vi "Copy VIP File sub.vi"(0 "CLI in":refnum<class "CLI.lvclass">, 5 "Array of created files":path[](array[path]), 11 "error in (no error)":errorcluster) -> (4 "CLI out":refnum<class "CLI.lvclass">, 15 "error out":errorcluster)   [LabVIEW 2023]
doc: "Copy VIP File sub.vi\n----------------------------------------------\nCopies the created *.vip file to the public user's documents folder\n\nInputs:\n---------------------\n- CLI in : LabVIEW Class Instance; \n- error in (no error) : Cluster; \n- Array of created files : 1DArrayOfPath; \n\nOutputs:\n---------------------\n- CLI out : LabVIEW Class Instance; \n- error out : Cluster; \n\n----------------------------------------------\n6/1/2021 nina\nZühlke Engineering AG\nCH-8952 Schlieren\nwww.zuehlke.com"
uses:
  <vilib>/Wiresmith Technology/G CLI/CLI Class/CLI.lvclass
panel:
  # "Connector Pane"
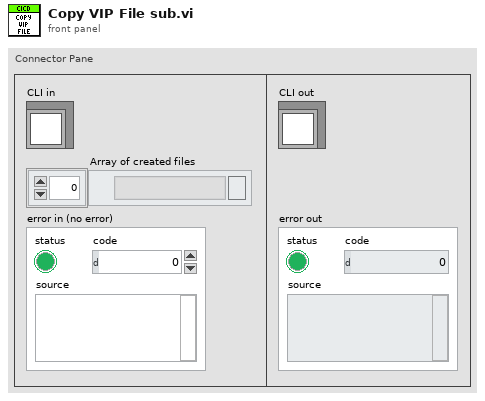
[diagram p1: front panel]
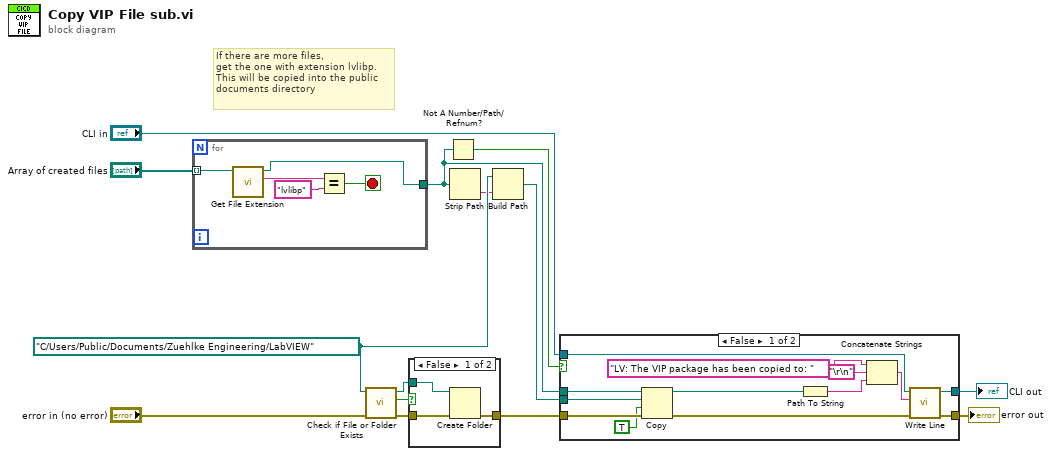
[diagram p0: block diagram]
diagram:
  w4 = path "C:/Users/Public/Documents/Zuehlke Engineering/LabVIEW" ("base path")
  # "If there are more files,\nget the one with extension lvlibp.\nThis will be copied into the public\ndocuments directory"
  n1 = for {
    tunnel: "Array of created files" -> [w19] mode=indexing
    tunnel: [w18] -> w12
    stop <- w15 stop-if-true
    n2 = call <vilib>:"Get File Extension.vi"("file"=w19) -> ("lowercase file extension"=w17:string, "dup file"=w18:path)  [unwired: 6 in, 3 out]
    n3 = Equal?(x=w17, y="lvlibp") -> (x = y?=w15:bool)
  }
  n4 = call <vilib>:"Check if File or Folder Exists.vi"("error in (no error)"="error in (no error)", "path"=w4) -> ("error out"=w6:errorcluster, "file or folder exists?"=w7:bool, "dup path"=w5:path)  [unwired: 7 in]
  n5 = case shown="False" w7 {
    tunnel: w5 -> [w22 _]
    tunnel: w6 -> [w21 w23]
    tunnel: [w20 w23] -> w10
    frame False {
      n6 = Create Folder(path (use dialog)=w22, error in=w21) -> (error out=w20:errorcluster)  [unwired: 1 in, 2 out]
    }
    frame True {
    }
  }
  n7 = Not A Number/Path/Refnum?(number/path/refnum=w12) -> (NaN/Path/Refnum?=w2:bool)
  n8 = Strip Path(path=w12) -> (name=w3:string)  [unwired: 1 out]
  n9 = Build Path(base path=w4, name or relative path=w3) -> (appended path=w11:path)
  n10 = case shown="False" w2 {
    tunnel: [w36 w38] -> w14
    tunnel: "CLI in" -> [w35 w38]
    tunnel: w12 -> [w33 _]
    tunnel: w11 -> [w32 _]
    tunnel: w10 -> [w31 w37]
    tunnel: [w24 w37] -> w1
    frame False {
      n11 = Copy(8:w31, 9:TRUE ("overwrite (F)"), 10:w32, 11:w33) -> (0:w34:errorcluster, 3:w29:path)  [unwired: 1 in, 1 out]
      n12 = Path To String(path=w29) -> (string=w28:string)
      n13 = Concatenate Strings("LV: The VIP package has been copied to: " ("string"), "\r\n", w28) -> (w30:string)
      n14 = call <vilib>:"Write Line.vi"("error in (no error)"=w34, "Text to Write"=w30, "CLI in"=w35) -> ("error out"=w24:errorcluster, "CLI out"=w36:refnum<class "CLI.lvclass">)  [unwired: 7 in]
    }
    frame True {
    }
  }
  "CLI out" <- w14
  "error out" <- w1
